vi "new one.vi"() -> ()   [LabVIEW 2015]
uses:
  <vilib>/Utility/NIReport.llb/Append Report Text (str wrap).vi
  <vilib>/Instr/_visa.llb/VISA Configure Serial Port (Instr).vi
  <vilib>/Utility/NIReport.llb/NI_report.lvclass
panel:
  out "Program name":string
  out "MAC ID":string
  out "SERIAL NUMBER":string
  out "STATUS":string
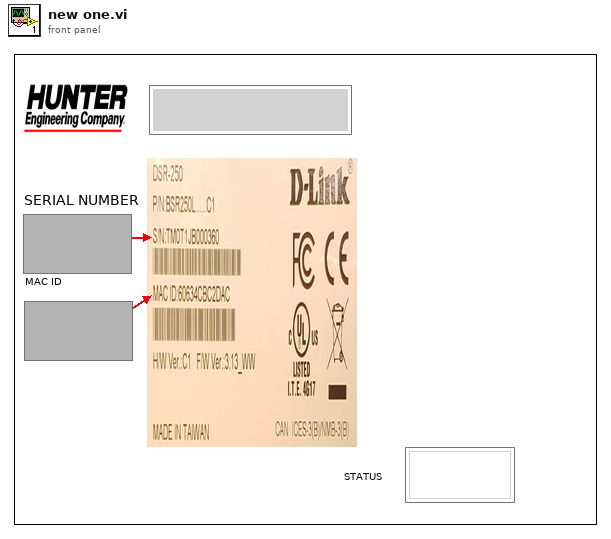
[diagram p1: front panel]
types:
  T1 = enum16{"Standard Report", "HTML", "Word", "Excel"}
  T2 = cluster{"Charset (-1)":i16, "Weight (-1)":i16, "Name":string, "Size":string}
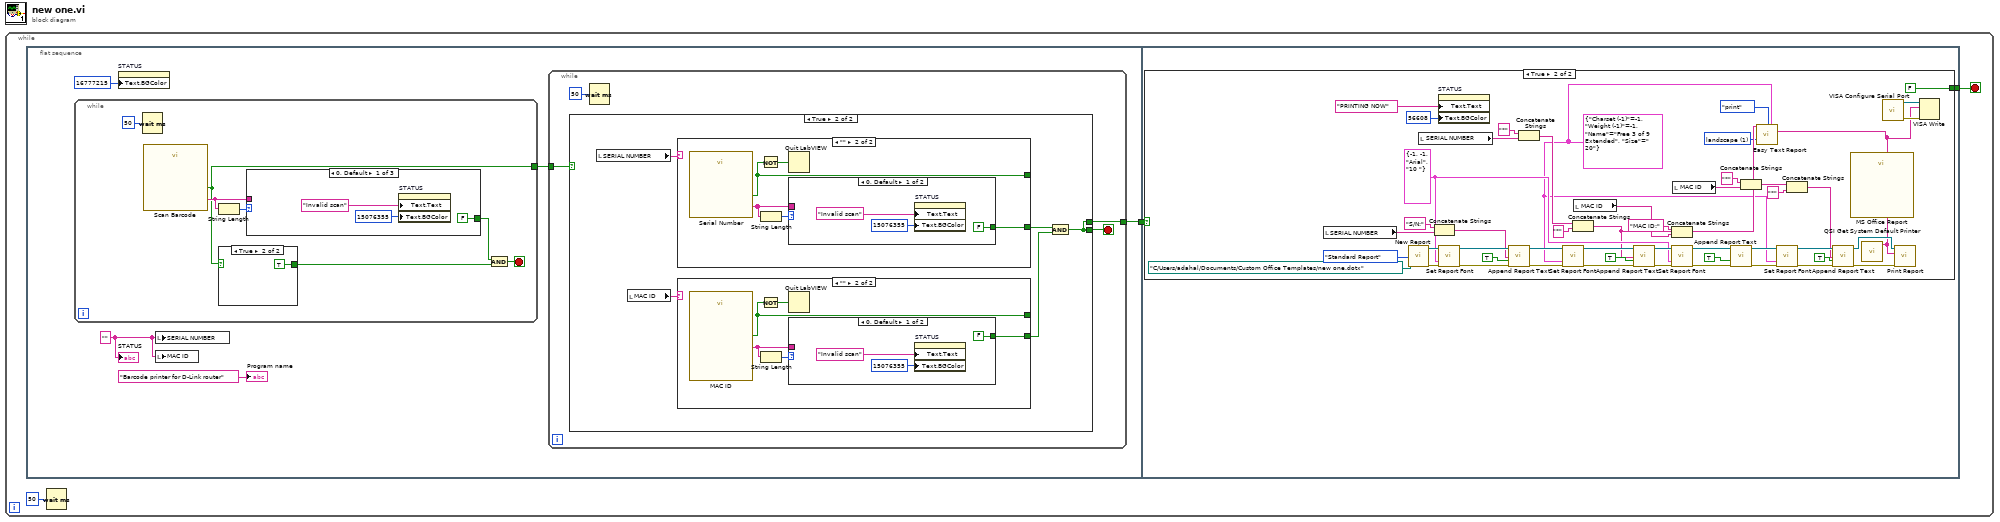
[diagram p0: block diagram]
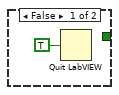
[diagram p2: hidden frame]
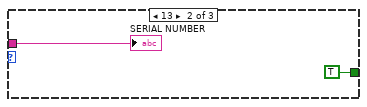
[diagram p3: hidden frame]
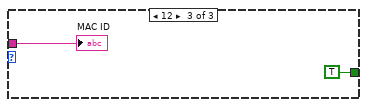
[diagram p4: hidden frame]
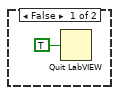
[diagram p5: hidden frame]
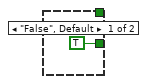
[diagram p6: hidden frame]
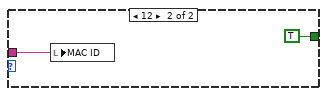
[diagram p7: hidden frame]
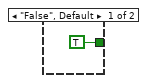
[diagram p8: hidden frame]
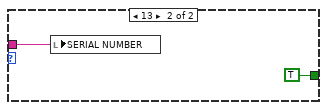
[diagram p9: hidden frame]
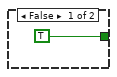
[diagram p10: hidden frame]
diagram:
  n1 = while {
    stop <- w2 stop-if-true
    n2 = flat-sequence {
      tunnel: [w6] -> w1
      tunnel: [w58] -> w2
      tunnel: w1 -> [w57]
      frame #0 {
        w7 = "" ("Serial Number")
        n3 = while {
          tunnel: [w13] -> w5
          stop <- w10 stop-if-true
          n4 = Wait (ms)(milliseconds to wait=u32 50) -> ()  [unwired: 1 out]
          n5 = call "Scan Barcode"() -> ("Scan now"=w15:string, "Submit"=w13:bool)  [unwired: 17 in, 1 out]
          n6 = String Length(string=w15) -> (length=w14:i32)
          n7 = case shown="True" w13 {
            tunnel: [_ TRUE] -> w11
            frame False {
              n8 = Quit LabVIEW(quit? (T)=TRUE) -> ()
            }
            frame True {
            }
          }
          n9 = case shown="0, Default" w14 {
            tunnel: w15 -> [_ w22 w24]
            tunnel: [FALSE TRUE TRUE] -> w12
            frame 0, Default {
              n10 = property on="STATUS" class="Str"("Text.Text"="Invalid scan", "Text.BGColor"=u32 15076355 ("Text.Text Colors:BG Color")) -> ()  [unwired: 2 in, 2 out]
            }
            frame 13 {
              "SERIAL NUMBER" <- w22
            }
            frame 12 {
              "MAC ID" <- w24
            }
          }
          n11 = And(x=w12, y=w11) -> (x .and. y?=w10:bool)
        }
        n12 = property on="STATUS" class="Str"("Text.BGColor"=u32 16777215 ("Text.Text Colors:BG Color")) -> ()  [unwired: 2 in, 2 out]
        n13 = local write "SERIAL NUMBER"(w7) -> ()
        n14 = local write "MAC ID"(w7) -> ()
        n15 = while {
          tunnel: w5 -> [w27]
          tunnel: [w26] -> w6
          stop <- w28 stop-if-true
          n16 = case shown="True" w27 {
            tunnel: [_ w30] -> w26
            tunnel: [_ w30] -> w28
            frame False {
              n17 = Quit LabVIEW(quit? (T)=TRUE) -> ()
            }
            frame True {
              n18 = local read "SERIAL NUMBER"() -> (w34:string)
              n19 = local read "MAC ID"() -> (w33:string)
              n20 = case shown="\"\"" w34 {
                tunnel: [TRUE w49] -> w32
                tunnel: [_ w47] -> _
                frame "False", Default {
                }
                frame "" {
                  n21 = call "Serial Number"() -> ("Serial Number"=w50:string, "Submit"=w47:bool)  [unwired: 17 in, 1 out]
                  n22 = Not(x=w47) -> (.not. x?=w48:bool)
                  n23 = String Length(string=w50) -> (length=w51:i32)
                  n24 = Quit LabVIEW(quit? (T)=w48) -> ()
                  n25 = case shown="0, Default" w51 {
                    tunnel: w50 -> [_ w56]
                    tunnel: [FALSE TRUE] -> w49
                    frame 0, Default {
                      n26 = property on="STATUS" class="Str"("Text.Text"="Invalid scan", "Text.BGColor"=u32 15076355 ("Text.Text Colors:BG Color")) -> ()  [unwired: 2 in, 2 out]
                    }
                    frame 13 {
                      n27 = local write "SERIAL NUMBER"(w56) -> ()
                    }
                  }
                }
              }
              n28 = case shown="\"\"" w33 {
                tunnel: [TRUE w38] -> w31
                tunnel: [_ w36] -> _
                frame "False", Default {
                }
                frame "" {
                  n29 = call "MAC ID"() -> ("Mac ID"=w40:string, "Submit"=w36:bool)  [unwired: 17 in, 1 out]
                  n30 = Not(x=w36) -> (.not. x?=w37:bool)
                  n31 = String Length(string=w40) -> (length=w39:i32)
                  n32 = Quit LabVIEW(quit? (T)=w37) -> ()
                  n33 = case shown="0, Default" w39 {
                    tunnel: w40 -> [_ w45]
                    tunnel: [FALSE TRUE] -> w38
                    frame 0, Default {
                      n34 = property on="STATUS" class="Str"("Text.Text"="Invalid scan", "Text.BGColor"=u32 15076355 ("Text.Text Colors:BG Color")) -> ()  [unwired: 2 in, 2 out]
                    }
                    frame 12 {
                      n35 = local write "MAC ID"(w45) -> ()
                    }
                  }
                }
              }
              n36 = And(x=w32, y=w31) -> (x .and. y?=w30:bool)
            }
          }
          n37 = Wait (ms)(milliseconds to wait=u32 50) -> ()  [unwired: 1 out]
        }
        "STATUS" <- w7
        "Program name" <- "Barcode printer for D-Link router" ("Program name")
      }
      frame #1 {
        n38 = case shown="True" w57 {
          tunnel: [TRUE FALSE] -> w58
          frame False {
          }
          frame True {
            w64 = u16 1 items=["portrait", "landscape"] ("orientation (portrait)")
            w63 = T2 {"Charset (-1)"=-1, "Weight (-1)"=-1, "Name"="Free 3 of 9 Extended", "Size"=" 20"} ("font settings")
            w90 = T2 {"Charset (-1)"=-1, "Weight (-1)"=-1, "Name"="Arial", "Size"="10 "} ("font settings")
            n39 = local read "SERIAL NUMBER"() -> (w70:string)
            n40 = call <vilib>:"New Report.vi"("report type"=T1."Standard Report", "template (empty)"=path "C:/Users/adahal/Documents/Custom Office Templates/new one.dotx") -> ("report out"=w108:refnum<class "NI_report.lvclass">, "error out"=w107:errorcluster)  [unwired: 12 in]
            n41 = local read "SERIAL NUMBER"() -> (w82:string)
            n42 = Concatenate Strings("S/N:" ("string"), w70) -> (w67:string)
            n43 = property on="STATUS" class="Str"("Text.Text"="PRINTING NOW" ("STATUS"), "Text.BGColor"=u32 56608 ("Text.Text Colors:BG Color")) -> ()  [unwired: 2 in, 2 out]
            n44 = call-dynamic "Set Report Font.vi"("report in"=w108, "font settings"=w90, "error in (no error)"=w107) -> ("report out"=w106:refnum<class "NI_report.lvclass">, "error out"=w105:errorcluster)  [unwired: 10 in, 1 out]
            n45 = call-poly <vilib>:"Append Report Text.vi"("report in"=w106, "text"=w67, "append on new line? (F)"=TRUE, "error in (no error)"=w105) -> ("report out"=w103:refnum<class "NI_report.lvclass">, "error out"=w102:errorcluster)  [unwired: 8 in, 2 out]
            n46 = Concatenate Strings("*" ("string"), w82) -> (w81:string)
            n47 = call-dynamic "Set Report Font.vi"("report in"=w103, "font settings"=w63, "error in (no error)"=w102) -> ("report out"=w100:refnum<class "NI_report.lvclass">, "error out"=w99:errorcluster)  [unwired: 10 in, 1 out]
            n48 = Concatenate Strings(w81, "*" ("string")) -> (w66:string)
            n49 = local read "MAC ID"() -> (w68:string)
            n50 = call-poly <vilib>:"Append Report Text.vi"("report in"=w100, "text"=w66, "append on new line? (F)"=TRUE, "error in (no error)"=w99) -> ("report out"=w91:refnum<class "NI_report.lvclass">, "error out"=w92:errorcluster)  [unwired: 8 in, 2 out]
            n51 = Concatenate Strings("MAC ID:" ("string"), w68) -> ()  [unwired: 1 out]
            n52 = call-dynamic "Set Report Font.vi"("report in"=w91, "font settings"=w90, "error in (no error)"=w92) -> ("report out"=w93:refnum<class "NI_report.lvclass">, "error out"=w95:errorcluster)  [unwired: 10 in, 1 out]
            n53 = local read "MAC ID"() -> (w77:string)
            n54 = call-poly <vilib>:"Append Report Text.vi"("report in"=w93, "append on new line? (F)"=TRUE, "error in (no error)"=w95) -> ("report out"=w86:refnum<class "NI_report.lvclass">, "error out"=w87:errorcluster)  [unwired: 9 in, 2 out]
            n55 = Concatenate Strings("*" ("string"), w77) -> (w78:string)
            n56 = call-dynamic "Set Report Font.vi"("report in"=w86, "font settings"=w63, "error in (no error)"=w87) -> ("report out"=w85:refnum<class "NI_report.lvclass">, "error out"=w88:errorcluster)  [unwired: 10 in, 1 out]
            n57 = Concatenate Strings(w78, "*" ("string")) -> (w75:string)
            n58 = call-poly <vilib>:"Append Report Text.vi"("report in"=w85, "text"=w75, "append on new line? (F)"=TRUE, "error in (no error)"=w88) -> ("report out"=w69:refnum<class "NI_report.lvclass">, "error out"=w84:errorcluster)  [unwired: 8 in, 2 out]
            n59 = call "MS Office Report"() -> ()  [unwired: 27 in, 1 out]
            n60 = call "QSI Get System Default Printer.vi"() -> ("System Default Printer"=w60:string)  [unwired: 4 in, 1 out]
            n61 = call <vilib>:"Easy Text Report.vi"("text to be printed"=w66, "print or save? (Word/Excel/HTML)"=enum16{"print", "save"}."print", "font settings"=w63, "printer name (default) or file path (dialog)"=w60, "orientation (portrait)"=w64) -> ()  [unwired: 10 in, 1 out]
            n62 = call-poly "VISA Configure Serial Port"() -> ("VISA resource name out"=w61:refnum<visa-resource-name>, "error out"=w62:errorcluster)  [unwired: 14 in]
            n63 = call-dynamic "Print Report.vi"("report in"=w69, "printer name (default)"=w60, "error in (no error)"=w84) -> ()  [unwired: 11 in, 2 out]
            n64 = VISA Write(VISA resource name=w61, write buffer=w60, error in (no error)=w62) -> ()  [unwired: 3 out]
          }
        }
      }
    }
    n65 = Wait (ms)(milliseconds to wait=u32 50) -> ()  [unwired: 1 out]
  }
